vi "WILT Read Cool Down Periods.vi"(8 "Error In":errorcluster, 11 "Input Cool Down Data":string[](array[string])) -> (0 "Error Out":errorcluster, 1 "Drying Time (Min)":dbl[](array[numeric]), 2 "Station Timeout Values (1-56) Seconds":dbl[](array[numeric]), 3 "Station Timeout Values":string)   [LabVIEW 2016]
panel:
  # "This is how I determine if the dryer \nshould re-inject water. I am expecting a dry\ntime of 90 min. If its less than a percentage of \nthis value. It will not re-inject"
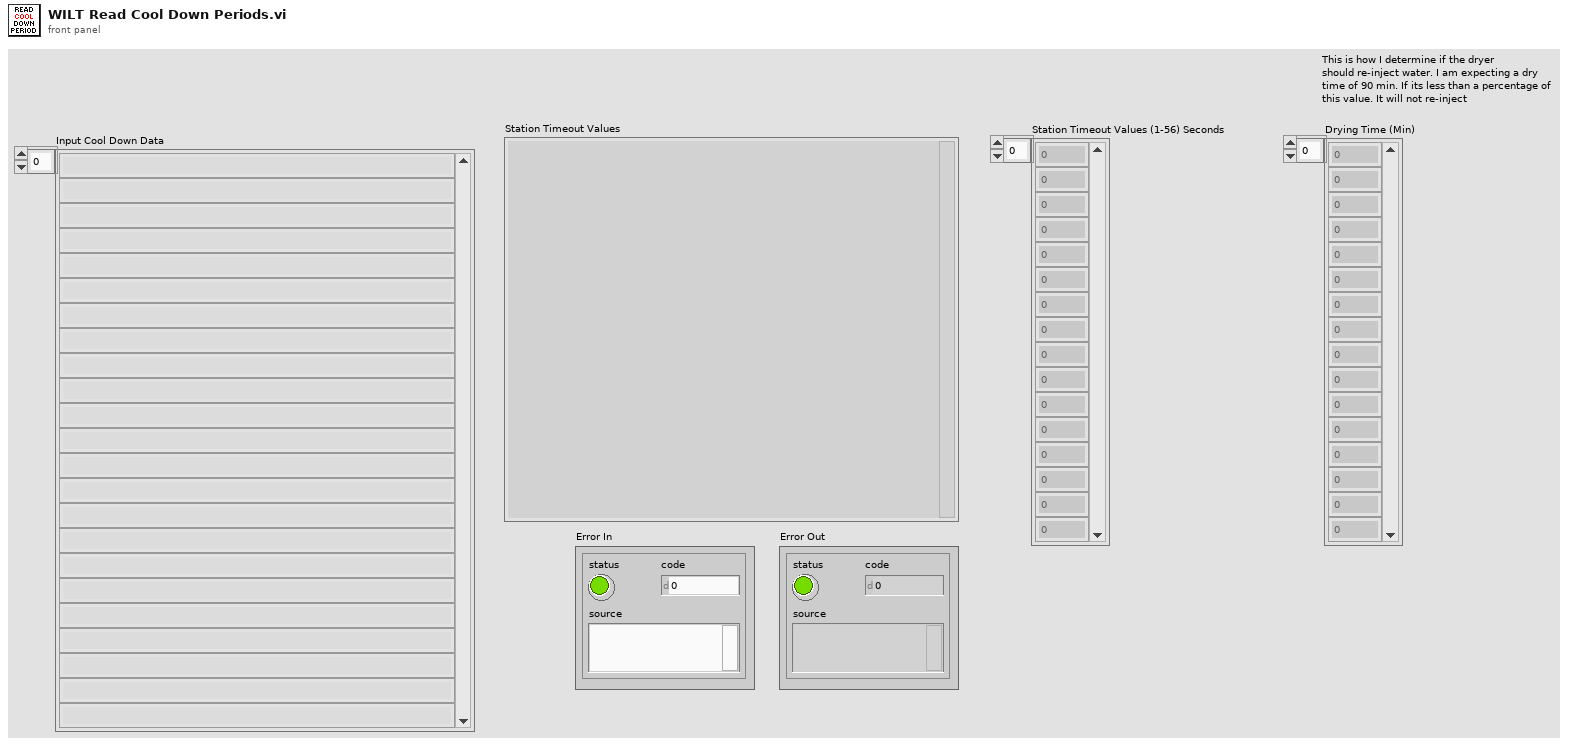
[diagram p1: front panel]
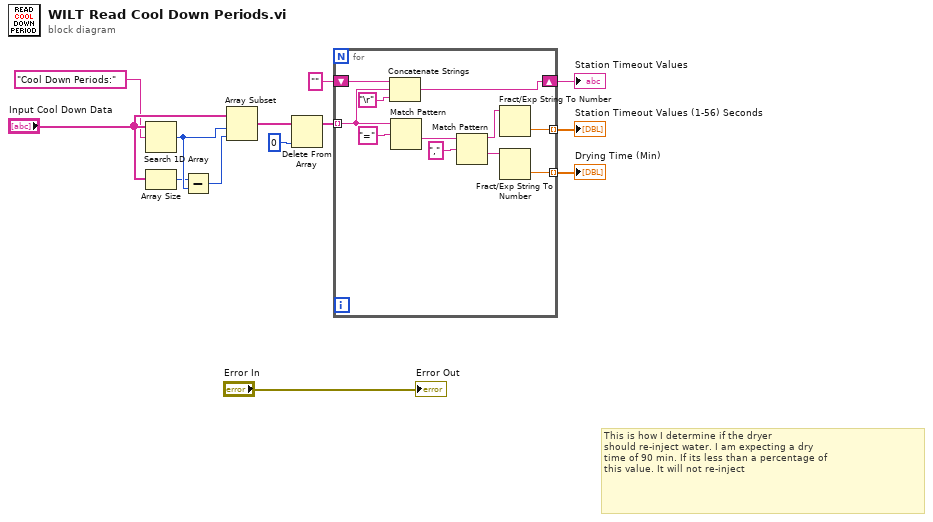
[diagram p0: block diagram]
diagram:
  # "This is how I determine if the dryer \nshould re-inject water. I am expecting a dry\ntime of 90 min. If its less than a percentage of \nthis value. It will not re-inject"
  n1 = Search 1D Array(1D array="Input Cool Down Data", element="Cool Down Periods:") -> (index of element=w7:i32)  [unwired: 1 in]
  n2 = Array Size(array="Input Cool Down Data") -> (size(s)=w3:i32)
  n3 = Subtract(x=w3, y=w7) -> (x-y=w4:i32)
  n4 = Array Subset(array="Input Cool Down Data", index=w7, length=w4) -> (w8:string[])
  n5 = Delete From Array(array=w8, index=0) -> (array with subset deleted=w10:string[])  [unwired: 1 in, 1 out]
  n6 = for {
    tunnel: w10 -> [w21] mode=indexing
    shift-right: [w22] -> w6
    shift-left: "" -> [w23]
    tunnel: [w19] -> w11 mode=indexing
    tunnel: [w14] -> w13 mode=indexing
    n7 = Concatenate Strings(w23, w21, "\r") -> (w22:string)
    n8 = Match Pattern(string=w21, regular expression="=") -> (after substring=w18:string)  [unwired: 1 in, 3 out]
    n9 = Match Pattern(string=w18, regular expression=",") -> (before substring=w16:string, after substring=w15:string)  [unwired: 1 in, 2 out]
    n10 = Fract/Exp String To Number(string=w16) -> (number=w19:dbl)  [unwired: 3 in, 1 out]
    n11 = Fract/Exp String To Number(string=w15) -> (number=w14:dbl)  [unwired: 3 in, 1 out]
  }
  "Station Timeout Values" <- w6
  "Station Timeout Values (1-56) Seconds" <- w11
  "Drying Time (Min)" <- w13
  "Error Out" <- "Error In"
